vi "CRYWindow LIB.vi"(10 "nData":i32, 11 "sAction":string) -> (2 "sData_Out":string)   [LabVIEW 2013]
uses:
  DataView/VIEW/CRYView Global.vi
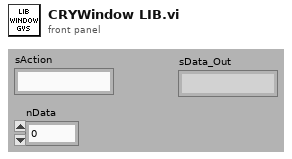
[diagram p1: front panel]
types:
  T1 = cluster{"sAction":string, "sData":string, "nData":i32, "pVIRef":refnum<vi>}
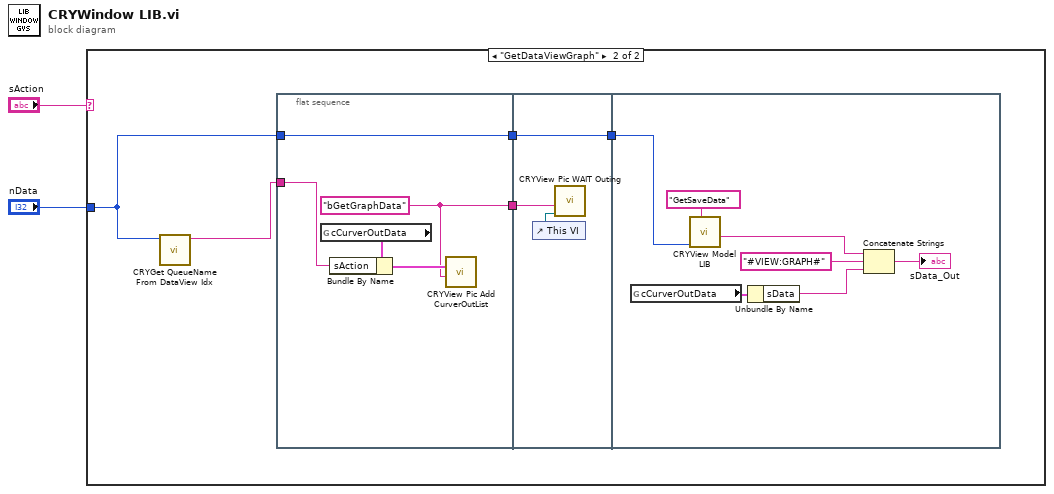
[diagram p0: block diagram]
diagram:
  n1 = case shown="\"GetDataViewGraph\"" "sAction" {
    tunnel: "nData" -> [_ w4]
    frame "False", Default {
    }
    frame "GetDataViewGraph" {
      n2 = call "CRYGet QueueName From DataView Idx.vi"("DataView Idx"=w4) -> ("DataView sQueueName"=w3:string)  [unwired: 10 in]
      n3 = flat-sequence {
        tunnel: w3 -> [w12]
        tunnel: w4 -> [w11]
        tunnel: [w11] -> w7
        tunnel: [w8] -> w5
        tunnel: w7 -> [w15]
        tunnel: [w15] -> w6
        tunnel: w5 -> [w13]
        tunnel: w6 -> [w21]
        frame #0 {
          w8 = "bGetGraphData" ("Label Name")
          n4 = global read "CRYView Global.vi" "cCurverOutData"() -> (w10:T1)
          n5 = Bundle By Name(cluster=w10, "sAction"=w12) -> (w9:T1)
          n6 = call "CRYView Pic Add CurverOutList.vi"("sName"=w8, "cCurverOutData"=w9) -> ()  [unwired: 10 in]
        }
        frame #1 {
          n7 = control-ref of="This VI"() -> (w14:refnum<vi>)
          n8 = call "CRYView Pic WAIT Outing.vi"("pVIRef"=w14, "sData"=w13) -> ()  [unwired: 9 in, 1 out]
        }
        frame #2 {
          n9 = global read "CRYView Global.vi" "cCurverOutData"() -> (w20:T1)
          n10 = call "CRYView Model LIB.vi"("sAction"="GetSaveData", "nData"=w21) -> ("sData_Out"=w18:string)  [unwired: 7 in, 2 out]
          n11 = Unbundle By Name(w20) -> ("sData"=w19:string)
          n12 = Concatenate Strings(w18, "#VIEW:GRAPH#" ("regular expression"), w19) -> (→"sData_Out":string)
        }
      }
    }
  }
